vi "hwOperation_Stop DAQ.vi"(7 "hwType":string, 8 "error in":errorcluster, 11 "hwDriverRef in":T1) -> (0 "error out":errorcluster, 3 "hwDriverRef out":T1)   [LabVIEW 2016]
uses:
  QX/hw_QX_hwDriverRef.ctl
  C:/Users/CL/Desktop/ZcDAQprj0811/ZcDAQprj/Modules/DAQ-Device/Hardware Drivers/QX/HBM LabVIEW Driver/DLLs/Hbm.Api.Common.dll
  QX/HBM LabVIEW Driver/DLLs/Hbm.Api.Common.dll
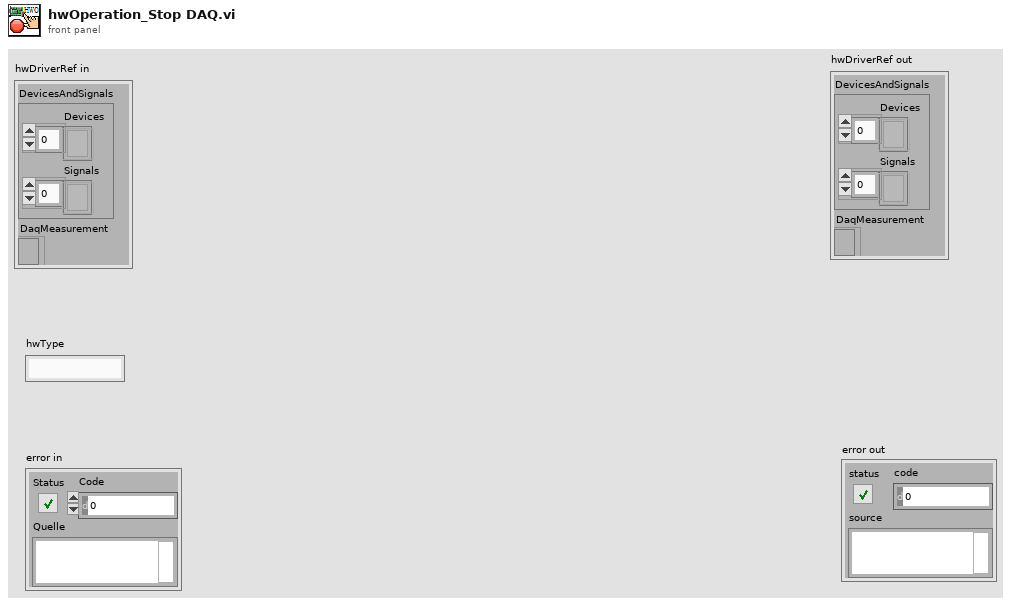
[diagram p1: front panel]
types:
  T1 = typedef "hw_QX_hwDriverRef.ctl" = cluster{"DevicesAndSignals":cluster{"Devices":refnum<k24>[], "Signals":refnum<k24>[]}, "DaqMeasurement":refnum<k24>}
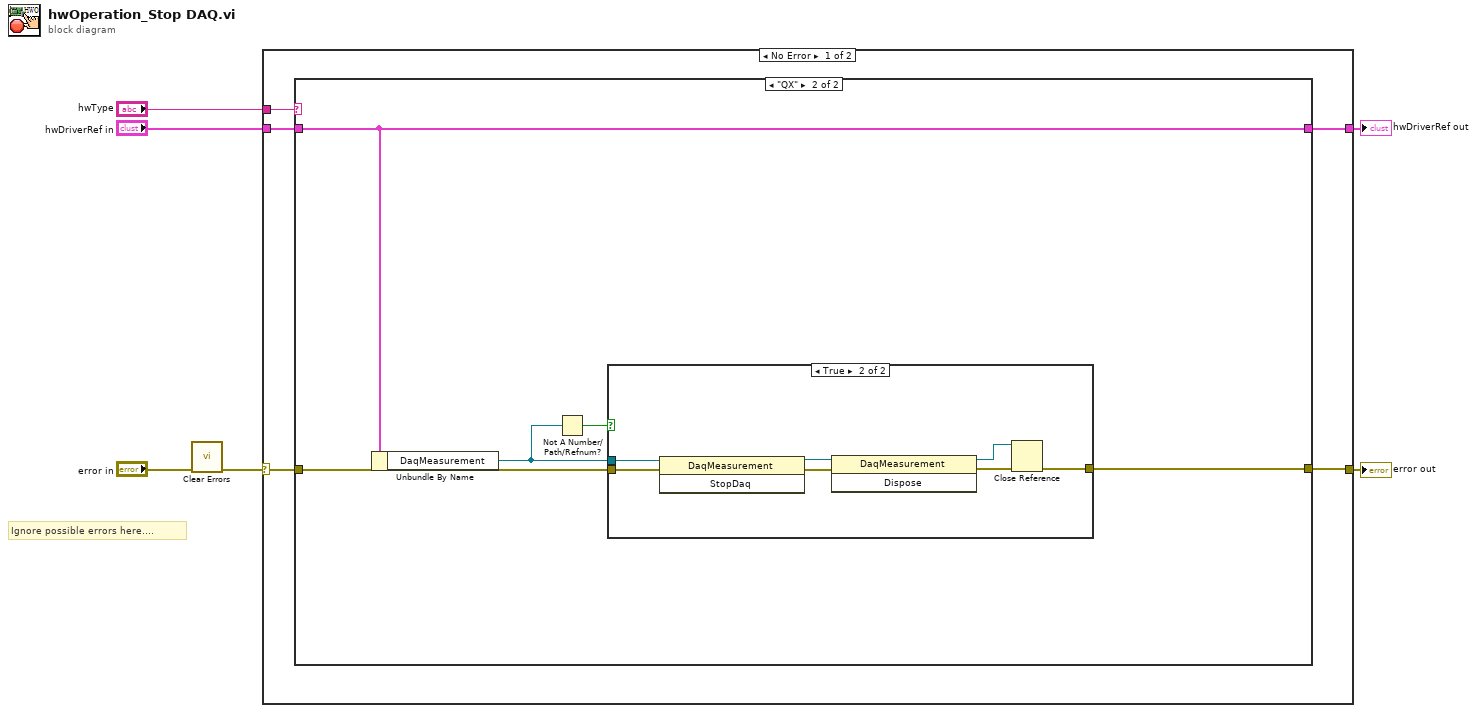
[diagram p0: block diagram]
diagram:
  # "Ignore possible errors here...."
  n1 = call <vilib>:"Clear Errors.vi"("error in (no error)"="error in") -> ("error out"=w1:errorcluster)  [unwired: 5 in, 1 out]
  n2 = case shown="No Error" w1 {
    selector: w1 -> [w10 w28]
    tunnel: [w11 w28] -> w5
    tunnel: "hwType" -> [w9 _]
    tunnel: "hwDriverRef in" -> [w8 w27]
    tunnel: [w7 w27] -> w2
    frame No Error {
      n3 = case shown="\"QX\"" w9 {
        tunnel: [w13 w16] -> w11
        tunnel: w10 -> [w13 w18]
        tunnel: w8 -> [w12 w17]
        tunnel: [w12 w17] -> w7
        frame "Simulation", Default {
        }
        frame "QX" {
          n4 = Unbundle By Name(w17) -> ("DaqMeasurement"=w15:refnum<k24>)
          n5 = Not A Number/Path/Refnum?(number/path/refnum=w15) -> (NaN/Path/Refnum?=w14:bool)
          n6 = case shown="True" w14 {
            tunnel: w18 -> [w19 w22]
            tunnel: [w19 w21] -> w16
            tunnel: w15 -> [_ w20]
            frame False {
            }
            frame True {
              n7 = invoke on="Methodenknoten" class="DaqMeasurement" method="StopDaq"(reference=w20, error in=w22) -> (reference out=w24:refnum<k24>, error out=w23:errorcluster)  [unwired: 1 in, 1 out]
              n8 = invoke on="Methodenknoten" class="DaqMeasurement" method="Dispose"(reference=w24, error in=w23) -> (reference out=w26:refnum<k24>, error out=w25:errorcluster)  [unwired: 1 in, 1 out]
              n9 = Close Reference(reference=w26, error in (no error)=w25) -> (error out=w21:errorcluster)
            }
          }
        }
      }
    }
    frame Error {
    }
  }
  "error out" <- w5
  "hwDriverRef out" <- w2
